vi "FPGA Frame Grabbing (Host).vi"(1 "Ctl Refnum":refnum<vi>) -> (0 "Image":T3(plugin-control))   [LabVIEW 2013, in "FPGA Frame Grabbing.lvlib"]
doc: "This is the host VI for the 10-Tap 8-Bit Camera with DRAM example. This example demonstrates how to acquire images from a 10-tap, 8-bit, extended configuration, Camera Link camera and display the images on the host. This example supports area scan and line scan cameras for both continuous and finite acquisitions.\n\nThis example also demonstrates the use of DRAM as a frame buffer for very high speed acquisitions. Data packing and flow-control are also employed to maximize use of the available DRAM and FIFOs in terms of both memory space and performance.\n\nAdditionally, the example demonstrates the serial server, which allows third-party camera configuration utilities to communicate with the camera using the Camera Link serial interface while this VI is running."
uses:
  FPGA Frame Grabbing.lvlib
  <vilib>/userdefined/High Color/nirio_resource_hc.ctl
  <vilib>/rvi/interface/common/niFpgaWaitOnOcc.vi
  <vilib>/FPGAPlugInAG/PCIe-1473R/niLvFpga_Open_PCIe-1473R.vi
  <vilib>/rvi/interface/common/dynamic/niFpgaDynamicAddResources.vi
  <vilib>/FPGAPlugInAG/Dynamic/niLvFpga_Reset_Dynamic.vi
  <vilib>/Utility/error.llb/Error Cluster From Error Code.vi
  <vilib>/rvi/errors/niLvFpgaAdjustHostInterfaceError.vi
  <vilib>/FPGAPlugInAG/Dynamic/niLvFpga_Run_Dynamic.vi
  <vilib>/FPGAPlugInAG/Dynamic/niLvFpga_Close_Dynamic.vi
  <vilib>/rvi/interface/nirviOpenFPGA/nirviOpenFPGA.xnode
  LabVIEW/Vision/Vision-RIO/Vision-RIO/10-Tap 8-bit Camera with DRAM/FPGA Bitfiles/10-Tap8-bitwith_DRAM.lvbitx
  <vilib>/rvi/interface/nirviMethod/nirviMethod.xnode
  <vilib>/rvi/interface/nirviReadWriteControl/nirviReadWriteControl.xnode
  <vilib>/rvi/interface/nirviCloseFPGA/nirviCloseFPGA.xnode
  NiFpgaLv.dll
  <vilib>/rvi/interface/Simulation/niFpgaSimulationCallBeginRW.vi
  <vilib>/rvi/errors/niLvFpgaMergeErrorWithErrorCode.vi
  <vilib>/FPGAPlugInAG/Dynamic/niLvFpga_ConfigureFifo_Dynamic.vi
  <vilib>/FPGAPlugInAG/Dynamic/niLvFpga_StartFifo_Dynamic.vi
  <vilib>/FPGAPlugInAG/Dynamic/niLvFpga_ReadFifo_Dynamic.vi
panel:
  in  "DMA Buffer Size\n(In Images)":u32=64 caption="DMA Buffer Size"
  in  "Signal Mapping":T1(ring)=enum."Basler 10-tap"
  out "Acq In Progress":bool
  in  "Line Scan":bool
  in  "Frames To Acquire":u32=1 caption="Frames To Acquire\n(0 = infinite)"
  in  "Cancel":bool
  out "Acq'd Frame Width":u32=2040
  in  "Stopped":bool=TRUE
  in  "RIO Device":T2="RIO0"
  out "DMA Write Timeout":bool
  in  "Start Serial Server":bool=TRUE
  out "Frames Acq'd":u32=1
  out "Acq'd Frame Height":u32=1088
  in  "Acquire":bool
  in  "Image Height":u32=1088 max=65535
  in  "Image Width":u32=2040 max=65535 step=40
  out "Initialized":bool
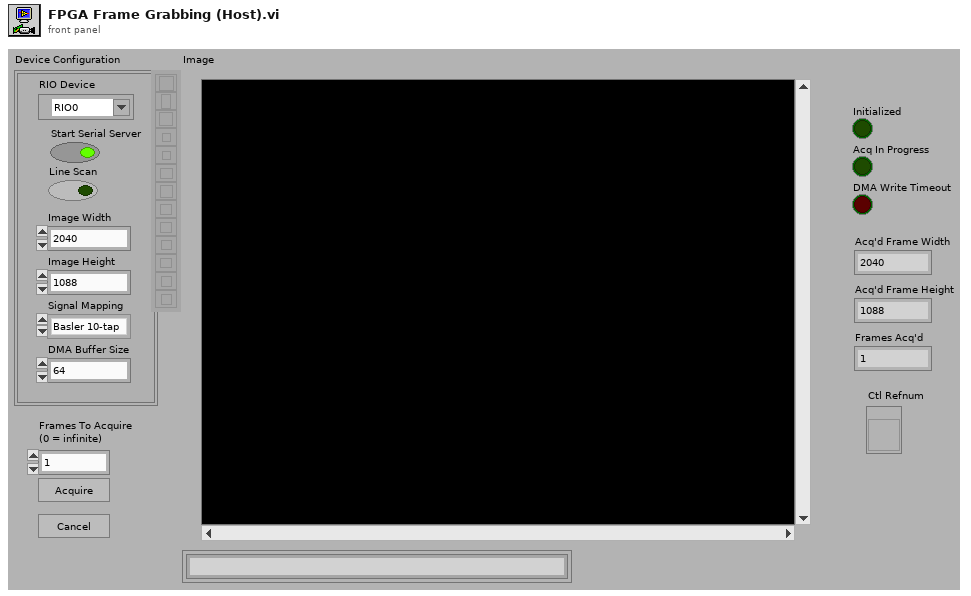
[diagram p1: front panel]
types:
  T1 = enum8{"Standard", "Basler 10-tap", "Vosskühler 10-tap"}
  T2 = typedef "nirio_resource_hc.ctl" = tag
  T3 = typedef "IMAQ Image.ctl" = refnum<image>
  T4 = typedef "Image Type" = u32
  T5 = enum16{"big-endian, network order", "native, host order", "little-endian"}
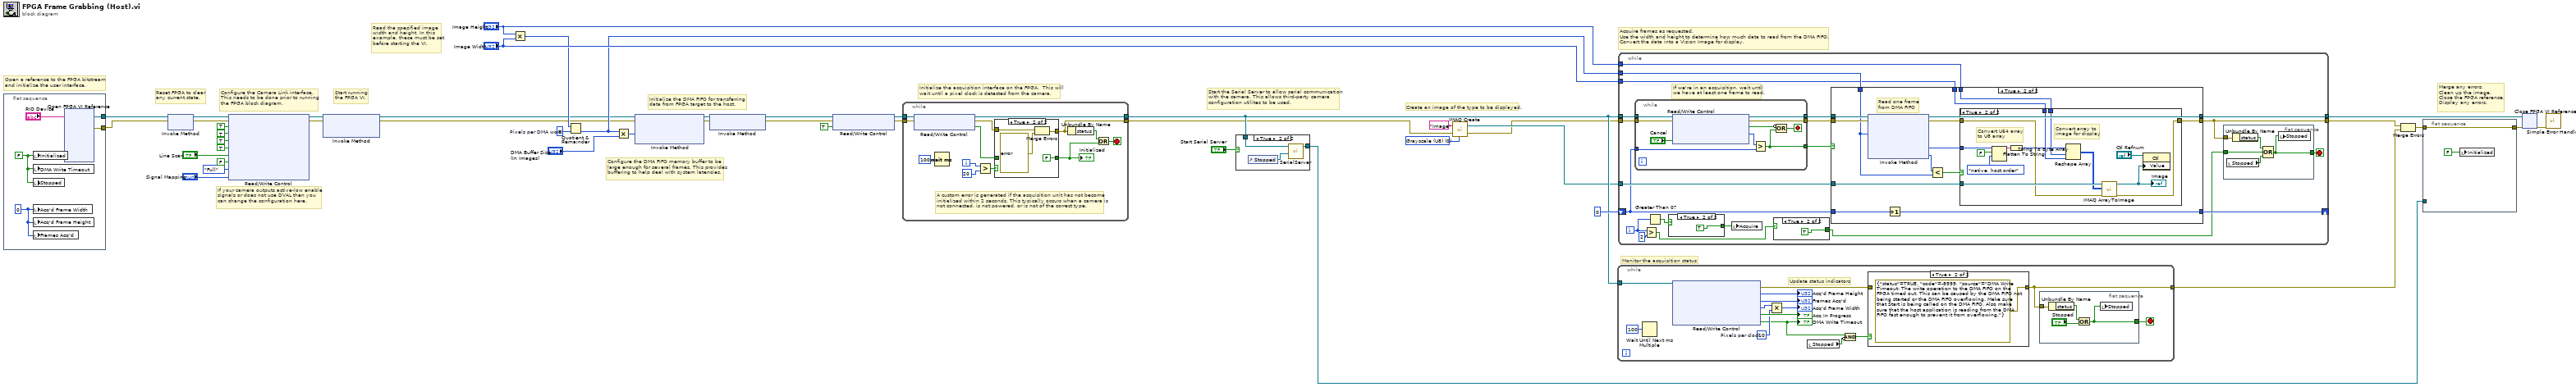
[diagram p0: block diagram]
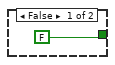
[diagram p4: hidden frame]
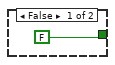
[diagram p5: hidden frame]
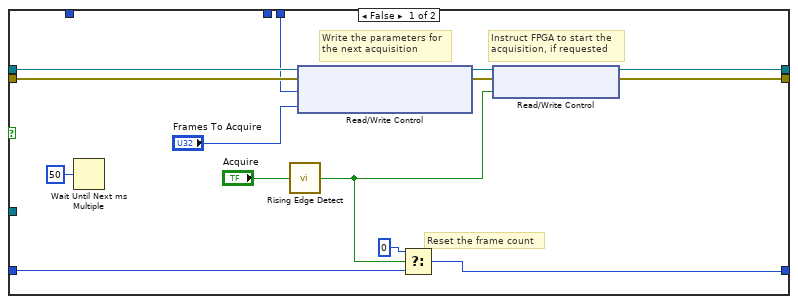
[diagram p6: hidden frame]
diagram:
  w5 = u32 8  # Pixels per DMA word
  w41 = T4 0 items=["Grayscale (U8)", "Grayscale (I16)", "Grayscale (SGL)", "Complex (CSG)", "RGB (U32)", "HSL (U32)", "RGB (U64)", "Grayscale (U16)"] ("Image Type")
  # "If your camera outputs active-low enable\nsignals or does not use DVAL then you \ncan change the configuration here."
  # "Configure the DMA FIFO memory buffer to be\nlarge enough for several frames. This provides\nbuffering to help deal with system latencies."
  # "Start running\nthe FPGA VI."
  # "Reset FPGA to clear\nany current state."
  # "Read the specified image\nwidth and height. In this\nexample, these must be set\nbefore starting the VI."
  # "Merge any errors.\nClean up the image.\nClose the FPGA reference.\nDisplay any errors."
  # "Acquire frames as requested.\nUse the width and height to determine how much data to read from the DMA FIFO.\nConvert the data into a Vision Image for display."
  # "Monitor the acquisition status"
  # "Start the Serial Server to allow serial communication\nwith the camera. This allows third-party camera\nconfiguration utilites to be used."
  # "Create an image of the type to be displayed."
  # "Initialize the acquisition interface on the FPGA.  This will\nwait until a pixel clock is detected from the camera."
  # "Initialize the DMA FIFO for transferring\ndata from FPGA target to the host."
  # "Configure the Camera Link interface.\nThis needs to be done prior to running\nthe FPGA block diagram."
  # "Open a reference to the FPGA bitstream\nand initialize the user interface."
  n1 = flat-sequence {
    tunnel: [w48] -> w33
    tunnel: [w47] -> w45
    frame #0 {
      w50 = u32 0 ("Num Lines Acq'd")
      w46 = FALSE ("stop")
      n2 = local write "Initialized"(w46) -> ()
      n3 = local write "DMA Write Timeout"(w46) -> ()
      n4 = local write "Stopped"(w46) -> ()
      n5 = local write "Acq'd Frame Width"(w50) -> ()
      n6 = local write "Acq'd Frame Height"(w50) -> ()
      n7 = local write "Frames Acq'd"(w50) -> ()
      n8 = xnode "Open FPGA VI Reference"("resource name"="RIO Device") -> ("FPGA VI Reference Out"=w48:refnum<k20>, "error out"=w47:errorcluster)  [unwired: 1 in]
    }
  }
  n9 = xnode "Invoke Method"("FPGA VI Reference In"=w33, "error in"=w45) -> ("FPGA VI Reference Out"=w22:refnum<k20>, "error out"=w25:errorcluster)
  n10 = xnode "Read/Write Control"("FPGA VI Reference In"=w22, "error in"=w25, "CL Config.FVAL Active High"=TRUE ("IO Module Config.CL FVAL Active High"), "CL Config.LVAL Active High"=TRUE ("IO Module Config.CL LVAL Active High"), "CL Config.DVAL Active High"=TRUE ("IO Module Config.CL DVAL Active High"), "CL Config.Spare Active High"=TRUE ("IO Module Config.CL Spare Active High"), "CL Config.Line Scan"="Line Scan", "Acq Control.Ignore DVAL"=FALSE ("CL Config.Line Scan"), "CL Config.Configuration"=enum8{"Base", "Medium", "Full"}."Full", "CL Config.Signal Mapping"="Signal Mapping") -> ("FPGA VI Reference Out"=w26:refnum<k20>, "error out"=w24:errorcluster)
  n11 = xnode "Invoke Method"("FPGA VI Reference In"=w26, "error in"=w24) -> ("FPGA VI Reference Out"=w2:refnum<k20>, "error out"=w1:errorcluster)  [unwired: 1 in]
  n12 = Multiply(x="Image Height", y="Image Width") -> (x*y=w4:u32)
  n13 = Quotient & Remainder(x=w4, y=w5) -> (floor(x/y)=w3:u32)  [unwired: 1 out]
  n14 = Multiply(x=w3, y="DMA Buffer Size\n(In Images)") -> (x*y=w16:u32)
  n15 = xnode "Invoke Method"("FPGA VI Reference In"=w2, "error in"=w1, "Requested Depth"=w16) -> ("FPGA VI Reference Out"=w32:refnum<k20>, "error out"=w31:errorcluster)  [unwired: 1 out]
  n16 = xnode "Invoke Method"("FPGA VI Reference In"=w32, "error in"=w31) -> ("FPGA VI Reference Out"=w17:refnum<k20>, "error out"=w30:errorcluster)
  n17 = xnode "Read/Write Control"("FPGA VI Reference In"=w17, "error in"=w30, "Acq Control.Initialize"=TRUE ("Arm Acquisition")) -> ("FPGA VI Reference Out"=w44:refnum<k20>, "error out"=w43:errorcluster)
  n18 = while {
    tunnel: w44 -> [w58]
    tunnel: w43 -> [w57]
    tunnel: [w56] -> w13
    tunnel: [w60] -> w12
    i -> [w52]
    stop <- w63 stop-if-true
    # "A custom error is generated if the acquisition unit has not become\ninitialized within 2 seconds. This typically occurs when a camera is\nnot connected, is not powered, or is not of the correct type."
    n19 = xnode "Read/Write Control"("FPGA VI Reference In"=w58, "error in"=w57) -> ("FPGA VI Reference Out"=w56:refnum<k20>, "error out"=w55:errorcluster, "Acq Status.Initialized"=w54:bool)
    n20 = Wait (ms)(milliseconds to wait=u32 100) -> ()  [unwired: 1 out]
    n21 = Greater?(x=w52, y=20) -> (0:w53:bool)
    n22 = case shown="True" w53 {
      tunnel: [w65 FALSE] -> w59
      tunnel: w54 -> [w65 _]
      tunnel: w55 -> [w64 w67]
      tunnel: [w64 w69] -> w60
      frame False {
      }
      frame True {
        n23 = Merge Errors(w67, errorcluster {"status"=TRUE, "code"=-8999, "source"="Acquisition Initialization: This error typically occurs when a camera is not properly connected, is not powered, or is not of the correct type."} ("error in")) -> (w69:errorcluster)
      }
    }
    "Initialized" <- w59
    n24 = Unbundle By Name(w60) -> ("status"=w62:bool)
    n25 = Or(x=w62, y=w59) -> (x .or. y?=w63:bool)
  }
  n26 = case shown="True" "Start Serial Server" {
    tunnel: [_ w70] -> w34
    tunnel: w13 -> [_ w71]
    frame False {
    }
    frame True {
      n27 = control-ref of="Stopped"() -> (w72:refnum<vi>)
      n28 = call "SerialServer.vi"("Stop Refnum"=w72, "FPGA VI Reference In"=w71) -> ("FPGA VI Reference Out"=w70:refnum<k20>)  [unwired: 5 in]
    }
  }
  n29 = call "IMAQ Create"("Image Name"="Image", "Image Type"=w41, "error in (no error)"=w12) -> ("New Image"=w9:T3, "error out"=w8:errorcluster)  [unwired: 2 in]
  n30 = while {
    tunnel: w13 -> [w83]
    tunnel: [w86] -> w27
    stop <- w85 stop-if-true
    w76 = u32 10  # Pixels per clock
    # "Update status indicators"
    n31 = Wait Until Next ms Multiple(millisecond multiple=u32 100) -> ()  [unwired: 1 out]
    n32 = xnode "Read/Write Control"("FPGA VI Reference In"=w83) -> ("error out"=w82:errorcluster, "Acq Status.Lines Per Frame"=→"Acq'd Frame Height":u32, "Acq Status.Frames Acq'd"=→"Frames Acq'd":u32, "Acq Status.Clocks Per Line"=w77:u32, "Acq Status.Acq In Progress"=→"Acq In Progress":bool, "Acq Status.DMA Write Timeout"=w74:bool)  [unwired: 1 in, 1 out]
    "DMA Write Timeout" <- w74
    n33 = Multiply(x=w77, y=w76) -> (x*y=→"Acq'd Frame Width":u32)
    n34 = local read "Stopped"() -> (w73:bool)
    n35 = Compound Arithmetic op=AND(w74, invert w73) -> (w75:bool)
    n36 = case shown="True" w75 {
      tunnel: w82 -> [w91 _]
      tunnel: [w91 errorcluster {"status"=TRUE, "code"=-8999, "source"="DMA Write Timeout: The write operation to the DMA FIFO on the FPGA timed out. This can be caused by the DMA FIFO not being started or the DMA FIFO overflowing. Make sure that Start is being called on the DMA FIFO. Also make sure that the host application is reading from the DMA FIFO fast enough to prevent it from overflowing."} ("error out")] -> w86
      frame False {
      }
      frame True {
      }
    }
    n37 = flat-sequence {
      tunnel: w86 -> [w90]
      tunnel: [w88] -> w85
      frame #0 {
        n38 = Unbundle By Name(w90) -> ("status"=w89:bool)
        n39 = Or(x=w89, y="Stopped") -> (x .or. y?=w88:bool)
        n40 = local write "Stopped"(w88) -> ()
      }
    }
  }
  n41 = while {
    tunnel: w13 -> [w105]
    tunnel: w8 -> [w104]
    tunnel: w3 -> [w112]
    tunnel: "Image Height" -> [w111]
    tunnel: "Image Width" -> [w110]
    tunnel: w9 -> [w109]
    tunnel: [w107] -> w28
    tunnel: [w108] -> w40
    shift-right: [w100] -> _
    shift-left: u32 0 -> [w99]
    i -> [w96]
    stop <- w106 stop-if-true
    # "If we're in an acquisition, wait until\nwe have at least one frame to read."
    n42 = while {
      tunnel: w105 -> [w123]
      tunnel: w104 -> [w122]
      tunnel: [w120] -> w103
      tunnel: [w121] -> w102
      tunnel: w99 -> [w126]
      tunnel: [w124] -> w101
      stop <- w125 stop-if-true
      n43 = xnode "Read/Write Control"("FPGA VI Reference In"=w123, "error in"=w122, "Acq Control.Cancel Acq"="Cancel") -> ("FPGA VI Reference Out"=w121:refnum<k20>, "error out"=w120:errorcluster, "Acq Status.Acq In Progress"=w119:bool, "Acq Status.Frames Acq'd"=w118:u32)
      n44 = Greater?(x=w118, y=w126) -> (0:w124:bool)
      n45 = Compound Arithmetic op=OR(invert w119, w124) -> (w125:bool)
    }
    n46 = Greater?(x=w96, y=2) -> (0:w94:bool)
    n47 = Greater Than 0?(x=w96) -> (x > 0?=w98:bool)
    n48 = case shown="True" w98 {
      tunnel: [FALSE ("Acquire") TRUE ("Acquire")] -> w97
      frame False {
      }
      frame True {
      }
    }
    n49 = local write "Acquire"(w97) -> ()
    n50 = case shown="True" w94 {
      tunnel: [FALSE ("Acquire") TRUE ("Acquire")] -> w93
      frame False {
      }
      frame True {
      }
    }
    n51 = case shown="True" w101 {
      tunnel: w102 -> [w142 w153]
      tunnel: w103 -> [w141 w152]
      tunnel: w112 -> [_ w146]
      tunnel: w111 -> [w135 w159]
      tunnel: w110 -> [_ w158]
      tunnel: w109 -> [_ w157]
      tunnel: [w137 w155] -> w107
      tunnel: [w140 w154] -> w108
      tunnel: w99 -> [w143 w151]
      tunnel: [w145 w150] -> w100
      frame False {
        # "Reset the frame count"
        # "Instruct FPGA to start the\nacquisition, if requested"
        # "Write the parameters for\nthe next acquisition"
        n52 = Wait Until Next ms Multiple(millisecond multiple=u32 50) -> ()  [unwired: 1 out]
        n53 = call "Rising Edge Detect.vi"("Input"="Acquire") -> ("Pulse"=w133:bool)  [unwired: 4 in]
        n54 = xnode "Read/Write Control"("FPGA VI Reference In"=w142, "error in"=w141, "Acq Control.Line Scan Height"=w135, "Acq Control.Frames To Acq"="Frames To Acquire") -> ("FPGA VI Reference Out"=w139:refnum<k20>, "error out"=w138:errorcluster)
        n55 = Select(t=u32 0, s=w133, f=w143) -> (s? t:f=w145:u32)
        n56 = xnode "Read/Write Control"("FPGA VI Reference In"=w139, "error in"=w138, "Acq Control.Acquire"=w133) -> ("FPGA VI Reference Out"=w140:refnum<k20>, "error out"=w137:errorcluster)
      }
      frame True {
        # "Read one frame\nfrom DMA FIFO"
        n57 = xnode "Invoke Method"("FPGA VI Reference In"=w153, "error in"=w152, "Number of Elements"=w146) -> ("FPGA VI Reference Out"=w154:refnum<k20>, "error out"=w156:errorcluster, "Data"=w149:u64[], "Elements Remaining"=w147:u32)  [unwired: 1 in]
        n58 = Increment(x=w151) -> (x+1=w150:u32)
        n59 = Less?(x=w147, y=w146) -> (x < y?=w148:bool)
        n60 = case shown="True" w148 {
          tunnel: w159 -> [_ w173]
          tunnel: w158 -> [_ w172]
          tunnel: w157 -> [_ w171]
          tunnel: w156 -> [w160 w170]
          tunnel: [w160 w169] -> w155
          tunnel: w149 -> [_ w166]
          frame False {
            # "Do not display the image if we're falling behind in the acquisition."
          }
          frame True {
            # "Convert U64 array\nto U8 array"
            # "Convert array to\nimage for display"
            n61 = Flatten To String(anything=w166, prepend array or string size? (T)=FALSE, byte order (0:big-endian, network order)=T5."native, host order") -> (data string=w164:string)  [unwired: 1 in, 2 out]
            n62 = String To Byte Array(string=w164) -> (unsigned byte array=w163:u8[])
            n63 = Reshape Array(w163, w173, w172) -> (w168:u8[][])
            n64 = call "IMAQ ArrayToImage"("error in (no error)"=w170, "Image Pixels (U8)"=w168, "Image"=w171) -> ("error out"=w169:errorcluster, "Image Out"=w161:T3)  [unwired: 7 in]
            "Image" <- w161
            n65 = property class="Ctl"(reference="Ctl Refnum", "Value"=w161) -> ()  [unwired: 1 in, 2 out]
          }
        }
      }
    }
    n66 = flat-sequence {
      tunnel: w107 -> [w130]
      tunnel: [w129] -> w106
      tunnel: w93 -> [w127]
      frame #0 {
        n67 = local read "Stopped"() -> (w128:bool)
        n68 = Unbundle By Name(w130) -> ("status"=w131:bool)
        n69 = Compound Arithmetic op=OR(w131, w127, w128) -> (w129:bool)
        n70 = local write "Stopped"(w129) -> ()
      }
    }
  }
  n71 = Merge Errors(w28, w27) -> (w29:errorcluster)
  n72 = flat-sequence {
    tunnel: w29 -> [w175]
    tunnel: [w175] -> w37
    tunnel: w34 -> [_]
    frame #0 {
      n73 = local write "Initialized"(FALSE ("Module Enabled")) -> ()
    }
  }
  n74 = xnode "Close FPGA VI Reference"("FPGA VI Reference In"=w40, "error in"=w37) -> ("error out"=w35:errorcluster)
  n75 = call <vilib>:"Simple Error Handler.vi"("error in (no error)"=w35) -> ()  [unwired: 4 in, 5 out]
